vi "reward_behavior_michelle_visjitter_conswinAdapt_enticefx_TSLogV2.vi"() -> ()   [LabVIEW 2019]
doc: "The myRIO Project template acquires acceleration data from the onboard accelerometer and displays the changes of acceleration values in a waveform chart."
uses:
  <vilib>/myRIO/Common/Instrument Driver Framework/Utilities/typedefs/Generic FPGA Reference.ctl
  <vilib>/myRIO/Common/Instrument Driver Framework/Utilities/typedefs/myRIO v1.0 Reference.ctl
  <vilib>/myRIO/Common/Instrument Driver Framework/Utilities/typedefs/Hardware Version Enum.ctl
  <vilib>/myRIO/Common/Instrument Driver Framework/Utilities/typedefs/myRIO Generic Hardware Reference.ctl
  <vilib>/userdefined/High Color/nirio_resource_hc.ctl
  <vilib>/myRIO/Common/Instrument Driver Framework/Utilities/vis/Is FPGA Ref Available.vi
  <vilib>/myRIO/Common/Instrument Driver Framework/myRIO v1.0/Encoder/typedefs/Encoder Signal Mode.ctl
  <vilib>/myRIO/Common/Instrument Driver Framework/myRIO v1.0/Encoder/typedefs/Encoder Channels Enum.ctl
  <vilib>/myRIO/Instrument Drivers/Onboard IO/Encoder/typedefs/Encoder Reference.ctl
  <vilib>/myRIO/Instrument Drivers/Onboard IO/Encoder/Encoder.lvlib
  <vilib>/myRIO/Instrument Drivers/Onboard IO/Encoder/vis/Read.vi
  <vilib>/myRIO/Common/Instrument Driver Framework/myRIO v1.0/Encoder/typedefs/Encoder Configuration v1.0.ctl
  <vilib>/myRIO/Common/Instrument Driver Framework/myRIO v1.0/Encoder/vis/myRIO v1.1 Open Encoder.vi
  <vilib>/myRIO/Common/Instrument Driver Framework/myRIO v1.0/Encoder/vis/myRIO v1.0 Configure Encoder.vi
  <vilib>/myRIO/Instrument Drivers/Onboard IO/Encoder/vis/myRIO Encoder Open.xnode
  <vilib>/myRIO/Express VI/Onboard IO/Encoder/Encoder Express VI.xnode
  <vilib>/myRIO/Express VI/Onboard IO/DI/DI Express VI.xnode
  <vilib>/myRIO/Instrument Drivers/Onboard IO/DIO/vis/Read.vi
  <vilib>/myRIO/Instrument Drivers/Onboard IO/DIO/DIO.lvlib
  <vilib>/myRIO/Common/Instrument Driver Framework/myRIO v1.0/DIO/typedefs/DIO Channels Enum.ctl
  <vilib>/myRIO/Common/Instrument Driver Framework/myRIO v1.0/DIO/typedefs/DIO Channels List.ctl
  <vilib>/myRIO/Instrument Drivers/Onboard IO/DIO/typedefs/DIO Reference.ctl
  <vilib>/myRIO/Instrument Drivers/Onboard IO/DIO/vis/myRIO DIO Open.xnode
  <vilib>/myRIO/Common/Instrument Driver Framework/myRIO v1.0/DIO/vis/myRIO v1.1 Open DIO.vi
  <vilib>/myRIO/Instrument Drivers/Onboard IO/DIO/vis/Write.vi
  <vilib>/myRIO/Express VI/Onboard IO/DO/DO Express VI.xnode
  <vilib>/Analysis/Matrix/Datatypes/RealMatrix.ctl
  <vilib>/Analysis/Matrix/NI_Matrix.lvlib
panel:
  out "TimeLag":dbl
  out "Lag2":dbl
  out "TestTime":dbl
  out "RewTS":dbl[][](array[numeric])
  out "ConsTS":dbl[][](array[numeric])
  out "LickTS":dbl[][](array[numeric])
  out "ContrastChoice":dbl
  out "Its":i32
  out "BurstCriteria":dbl
  out "LickBurst 2":bool
  out "LickBurst":bool
  out "Enticements":i32
  in  "Entice":bool
  out "Misses":i32
  out "GoAhead":bool
  out "TimeOutDuration":i32
  out "ActiveTime":dbl
  out "ConsumptionGo":bool=TRUE
  out "Consumption_Period":i32
  out "Watch_Display":bool=TRUE
  in  "Give reward":bool
  out "Timings":dbl[](array[numeric])
  out "ISI":dbl
  out "ISI start time":dbl
  out "Time_out":bool=TRUE
  out "Time since lick":dbl
  out "Time of last lick":dbl
  out "Rewarded trials":dbl[](array[numeric])
  out "Rewards":u16
  out "Active Trial":bool
  out "Array temp2":T1
  out "Stimuli Loaded":bool
  out "Stim_ID":dbl[](array[numeric])
  out "Reward_mat":dbl[](array[numeric])
  out "Reward":bool=TRUE
  out "Frame clock":i32
  out "Licks":u32
  out "Lick":bool
  out "Time":dbl
  out "Stop":bool
  in  "Frames to collect":u32
  out "Overflow?":bool
  out "Counter Value":i32
  out "Velocity":dbl
  out "Velocity Plot":dbl[](graph)
  out "Velocity array":dbl[](array[numeric])
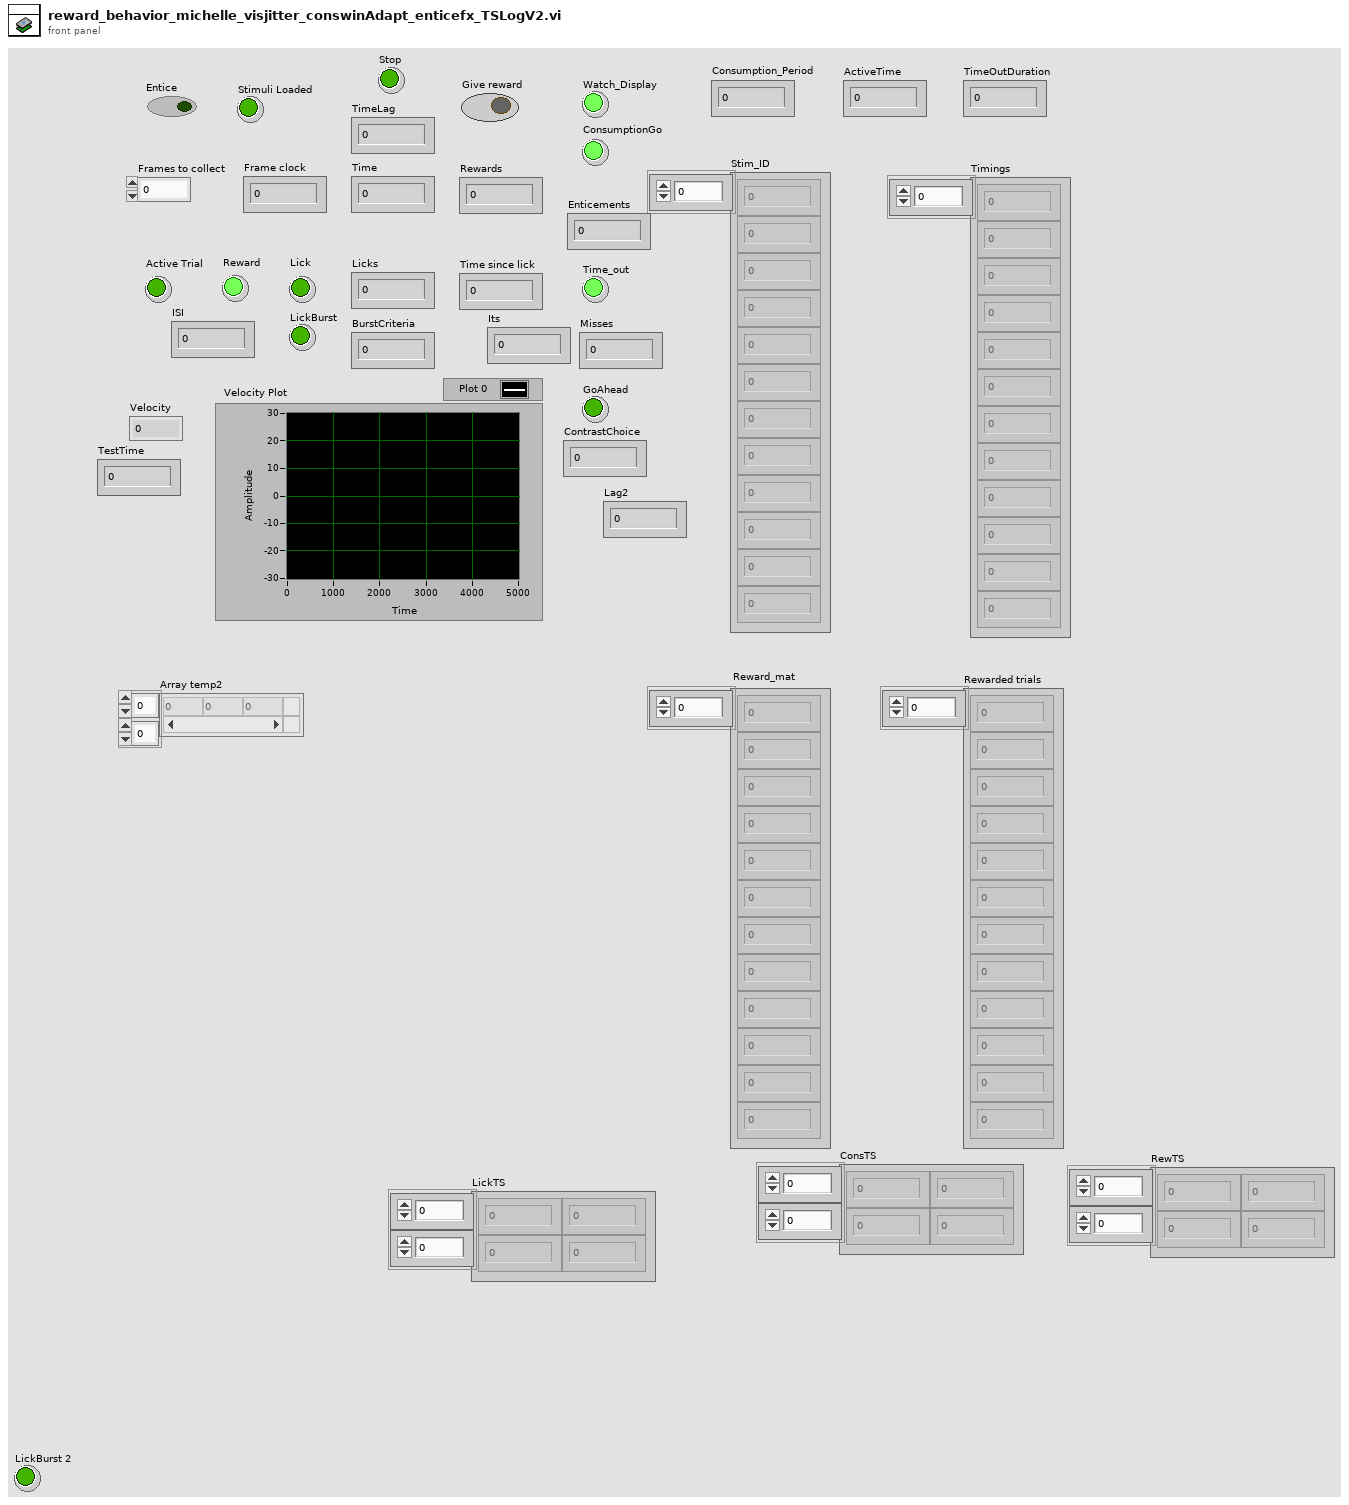
[diagram p1: front panel]
types:
  T1 = typedef "NI_Matrix.lvlib/RealMatrix.ctl" = dbl[][]
  T2 = typedef "Encoder.lvlib/Encoder Reference.ctl" = cluster{"myRIO Reference":T3, "Encoder Channels Enum":T7}
  T3 = typedef "myRIO Generic Hardware Reference.ctl" = cluster{"myRIO Model":T4, "myRIO Hardware Reference":T5}
  T4 = typedef "Hardware Version Enum.ctl" = enum16{"Unknown", "myRIO-1900", "myRIO-1950", "roboRIO", "NI ELVIS RIO CM", "ELVIS III"}
  T5 = typedef "myRIO v1.0 Reference.ctl" = cluster{"Generic FPGA Reference":T6, "Allow multiple opens":bool}
  T6 = typedef "Generic FPGA Reference.ctl" = refnum<k20>
  T7 = typedef "Encoder Channels Enum.ctl" = enum16{"Not Connected", "C/ENC0", "C/ENC1", "A/ENC", "A/ENC0", "A/ENC1", "A/ENC2", "A/ENC3", "A/ENC4", "A/ENC5", "A/ENC6", "A/ENC7", "A/ENC8", "A/ENC9", "B/ENC", "B/ENC0", "B/ENC1", "B/ENC2", "B/ENC3", "B/ENC4", "B/ENC5", "B/ENC6", "B/ENC7", "B/ENC8", "B/ENC9", "DIO/ENC0", "DIO/ENC1", "DIO/ENC2", "DIO/ENC3", "DIO/ENC4"}
  T8 = typedef "Encoder Signal Mode.ctl" = enum16{"Quadrature phase signal", "Step and direction signal"}
  T9 = typedef "nirio_resource_hc.ctl" = tag
  T10 = typedef "DIO.lvlib/DIO Reference.ctl" = cluster{"myRIO Reference":T3, "DIO Channels List":T11}
  T11 = typedef "DIO Channels List.ctl" = T12[]
  T12 = typedef "DIO Channels Enum.ctl" = enum16{"Not Connected", "C/DIO0", "C/DIO1", "C/DIO2", "C/DIO3", "C/DIO4", "C/DIO5", "C/DIO6", "C/DIO7", "A/DIO0", "A/DIO1", "A/DIO2", "A/DIO3", "A/DIO4", "A/DIO5", "A/DIO6", "A/DIO7", "A/DIO8", "A/DIO9", "A/DIO10", "A/DIO11", "A/DIO12", "A/DIO13", "A/DIO14", "A/DIO15", "A/DIO16", "A/DIO17", "A/DIO18", "A/DIO19", "B/DIO0", "B/DIO1", "B/DIO2", "B/DIO3", "B/DIO4", "B/DIO5", "B/DIO6", "B/DIO7", "B/DIO8", "B/DIO9", "B/DIO10", "B/DIO11", "B/DIO12", "B/DIO13", "B/DIO14", "B/DIO15", "B/DIO16", "B/DIO17", "B/DIO18", "B/DIO19", "LED0", "LED1", "LED2", "LED3", "Button0", "DIO/DIO0", "DIO/DIO1", "DIO/DIO2", "DIO/DIO3", "DIO/DIO4", "DIO/DIO5", "DIO/DIO6", "DIO/DIO7", "DIO/DIO8", "DIO/DIO9", "SPI/CS0", "SPI/CS1", "SPI/CS2", "SPI/CS3", "LED RADIO (Green)", "LED RADIO (Red)", "LED COMM (Green)", "LED COMM (Red)", "LED MODE (Green)", "LED MODE (Red)"}
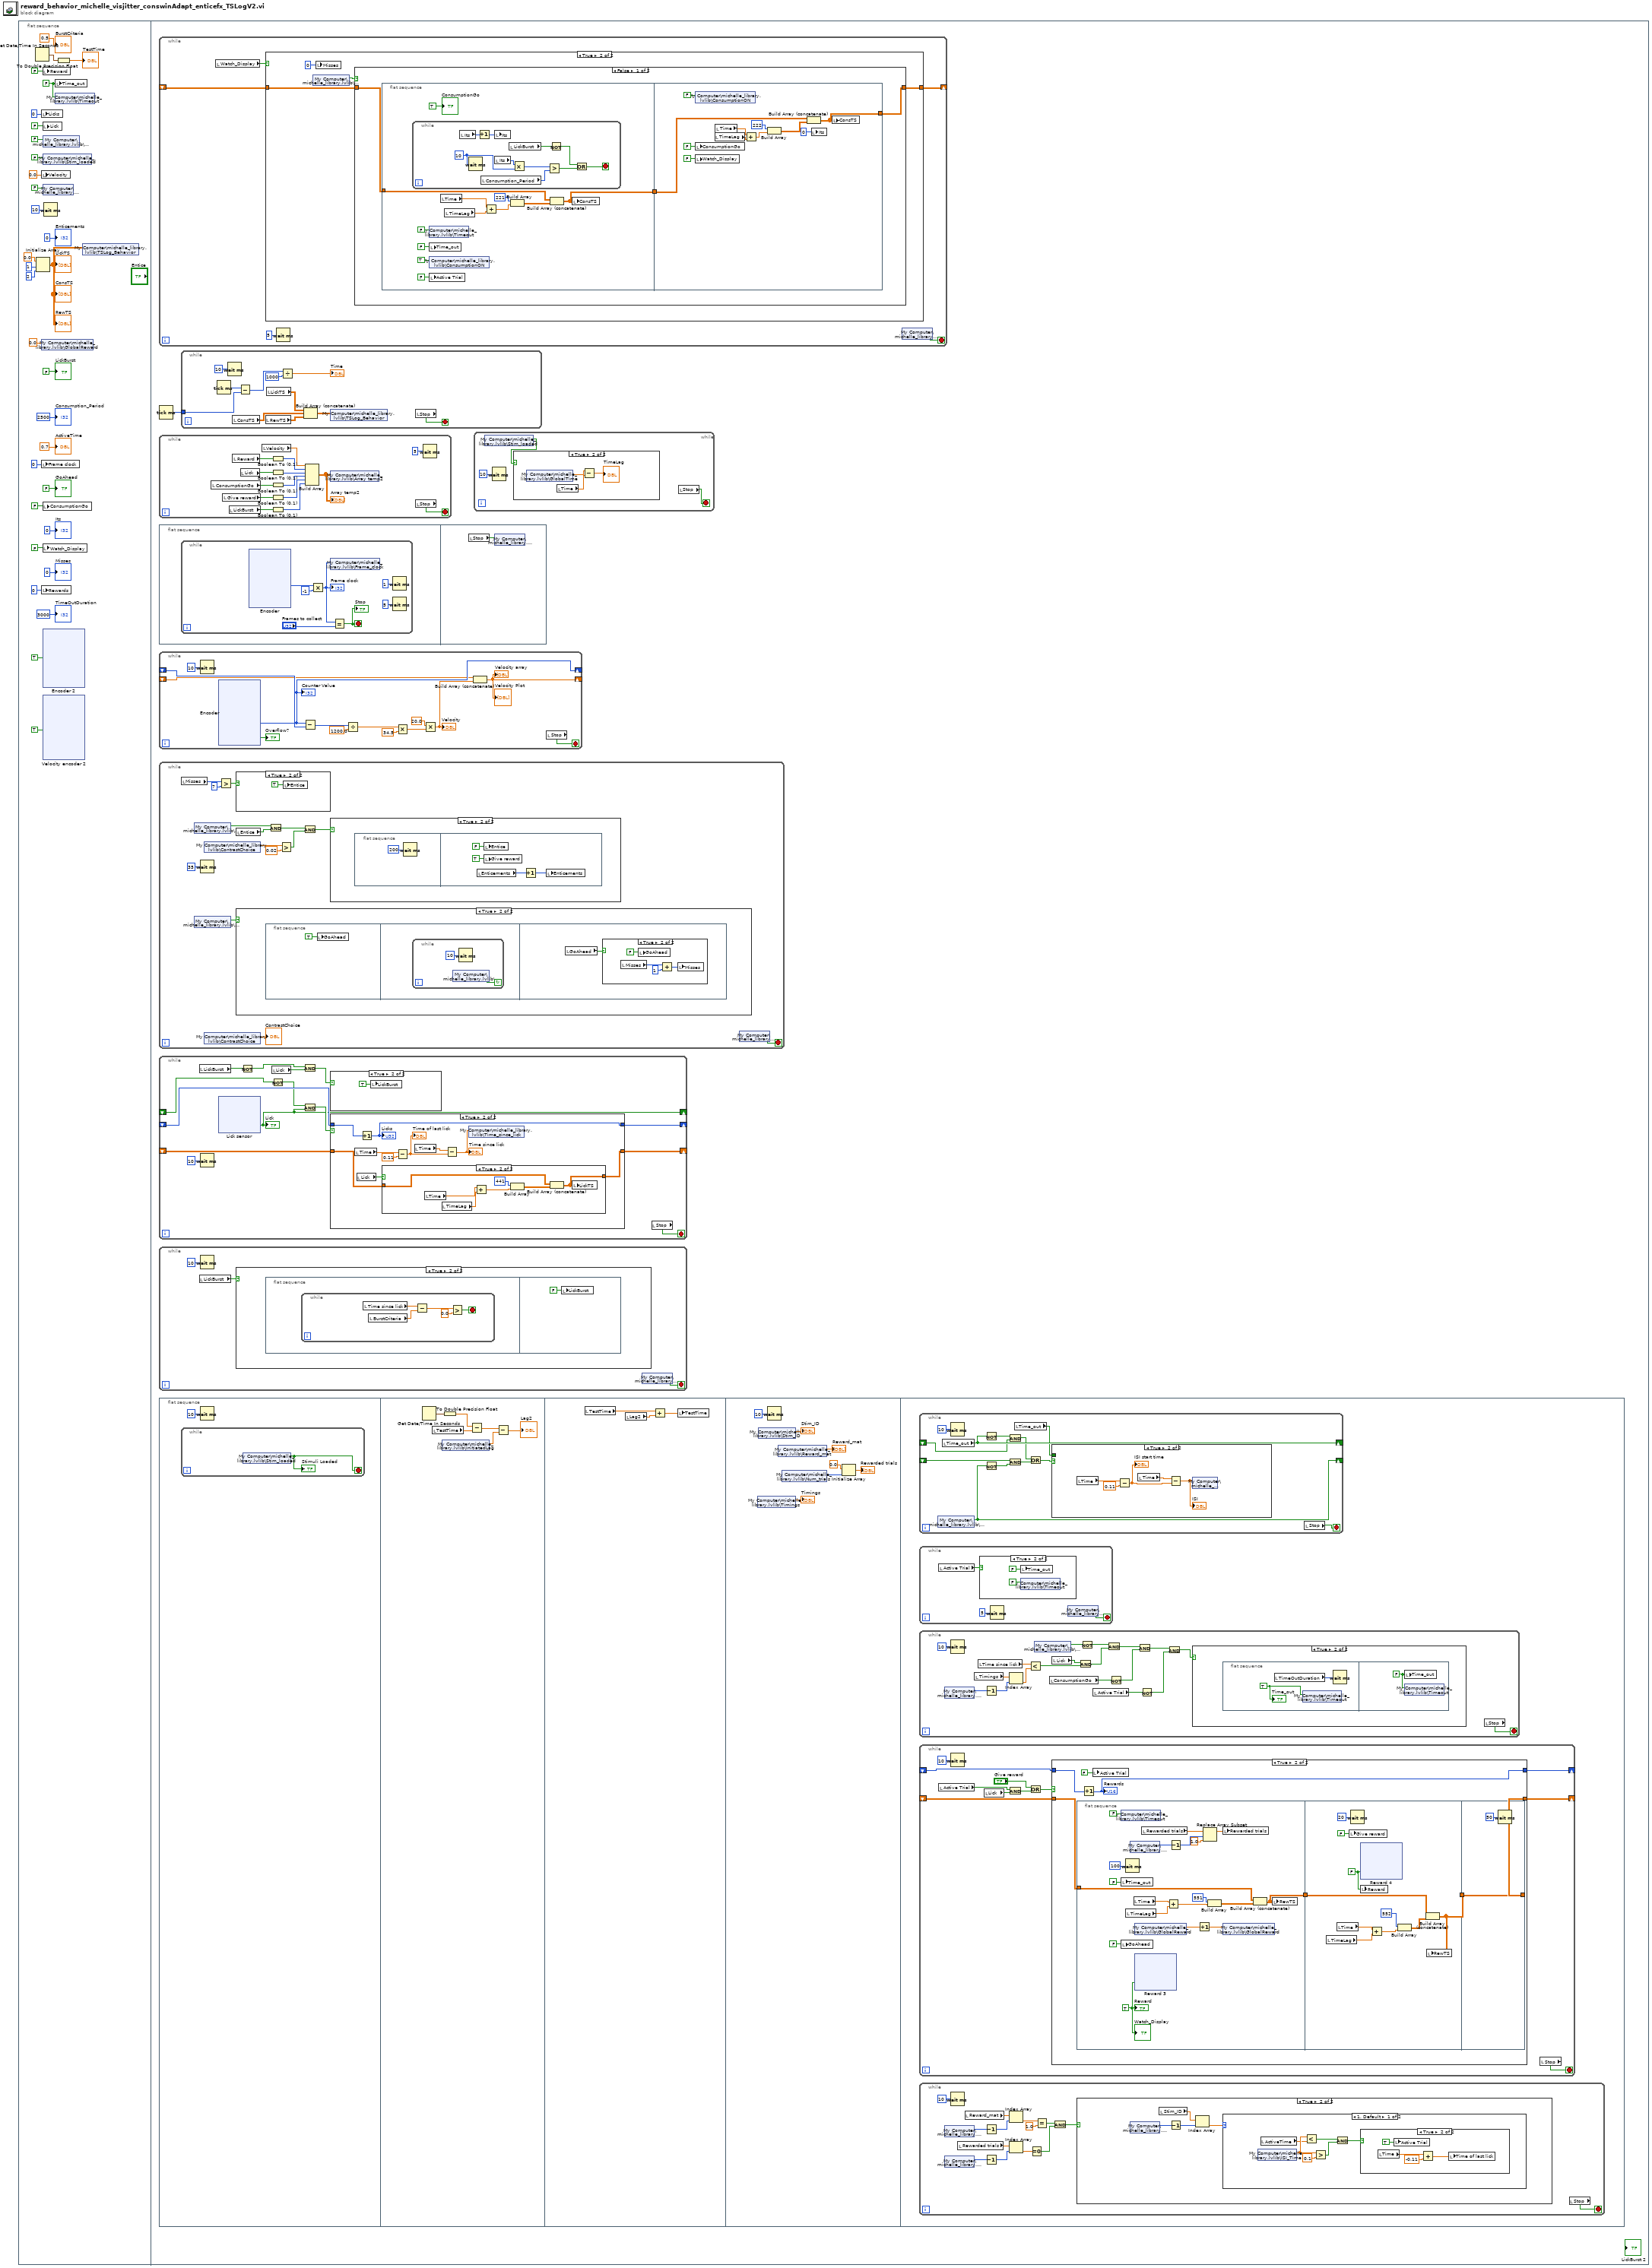
[diagram p0: block diagram]
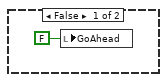
[diagram p6: hidden frame]
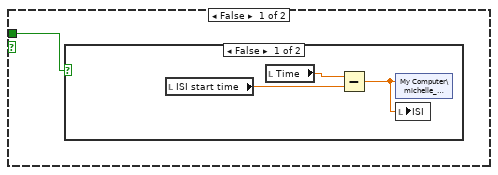
[diagram p12: hidden frame]
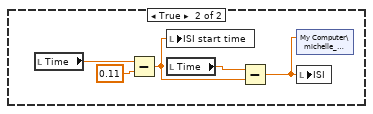
[diagram p13: hidden frame]
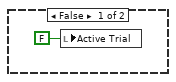
[diagram p14: hidden frame]
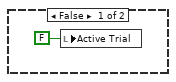
[diagram p15: hidden frame]
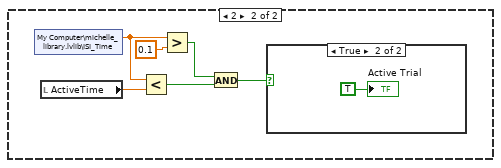
[diagram p16: hidden frame]
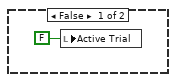
[diagram p17: hidden frame]
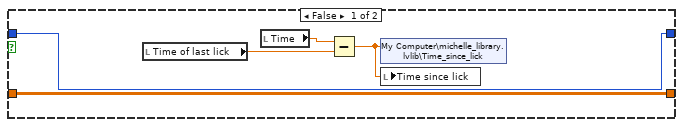
[diagram p20: hidden frame]
diagram:
  n1 = flat-sequence {
    frame #0 {
      w19 = FALSE ("Time_out")
      n2 = Get Date/Time In Seconds() -> (seconds since 1Jan1904=w3:timestamp)
      n3 = Initialize Array(0.0, 1, 2) -> (w1:dbl[][])
      "LickTS" <- w1
      "ConsTS" <- w1
      "RewTS" <- w1
      n4 = local write "Licks"(u32 0 ("Licks")) -> ()
      n5 = local write "Velocity"(0.0 ("Velocity")) -> ()
      n6 = shared-variable "My Computer\\michelle_library.lvlib\\GlobalReward"(0.0) -> ()  [unwired: 1 in, 1 out]
      n7 = local write "Frame clock"(u32 0 ("Frames")) -> ()
      n8 = local write "Rewards"(u16 0 ("Rewards")) -> ()
      n9 = local write "Reward"(FALSE ("Give reward")) -> ()
      n10 = local write "Lick"(FALSE ("Lick")) -> ()
      n11 = shared-variable "My Computer\\michelle_library.lvlib\\Display"(FALSE ("Display")) -> ()  [unwired: 1 in, 1 out]
      n12 = shared-variable "My Computer\\michelle_library.lvlib\\Stim_loaded"(FALSE ("Stim_loaded")) -> ()  [unwired: 1 in, 1 out]
      n13 = shared-variable "My Computer\\michelle_library.lvlib\\Stop"(FALSE ("Stop")) -> ()  [unwired: 1 in, 1 out]
      n14 = local write "ConsumptionGo"(FALSE ("ConsumptionGo")) -> ()
      n15 = local write "Watch_Display"(FALSE ("Watch_Display")) -> ()
      n16 = xnode "Encoder 2"("Reset Counter"=TRUE) -> ()  [unwired: 1 in, 4 out]
      n17 = xnode "Velocity encoder 2"("Reset Counter"=TRUE) -> ()  [unwired: 1 in, 4 out]
      n18 = Wait (ms)(milliseconds to wait=u32 10) -> ()  [unwired: 1 out]
      n19 = local write "Time_out"(w19) -> ()
      n20 = shared-variable "My Computer\\michelle_library.lvlib\\Timeout"(w19) -> ()  [unwired: 1 in, 1 out]
      n21 = To Double Precision Float(number=w3) -> (double precision float=→"TestTime":dbl)
      n22 = shared-variable "My Computer\\michelle_library.lvlib\\TSLog_Behavior"(w1) -> ()  [unwired: 1 in, 1 out]
      "Consumption_Period" <- 2500
      "ActiveTime" <- 0.7
      "TimeOutDuration" <- 3000
      "GoAhead" <- FALSE
      "Misses" <- 0
      "Enticements" <- 0
      "LickBurst" <- FALSE
      "BurstCriteria" <- 0.5
      "Its" <- 0
    }
    frame #1 {
      n23 = while {
        shift-right: [w169] -> _
        shift-left: _ -> [w170]
        stop <- w173 stop-if-true
        n24 = local read "Watch_Display"() -> (w172:bool)
        n25 = case shown="True" w172 {
          tunnel: w170 -> [w174 w176]
          tunnel: [w174 w175] -> w169
          frame False {
          }
          frame True {
            n26 = shared-variable "My Computer\\michelle_library.lvlib\\Display"() -> (w178:bool)  [unwired: 1 in, 1 out]
            n27 = local write "Misses"(0) -> ()
            n28 = case shown="False" w178 {
              tunnel: w176 -> [w181 w215]
              tunnel: [w179 w215] -> w175
              frame False {
                n29 = flat-sequence {
                  tunnel: w181 -> [w186]
                  tunnel: [w185] -> w180
                  tunnel: w180 -> [w209]
                  tunnel: [w208] -> w179
                  frame #0 {
                    n30 = while {
                      stop <- w197 stop-if-true
                      w198 = 10
                      n31 = local read "Its"() -> (w202:i32)
                      n32 = Wait (ms)(milliseconds to wait=w198) -> ()  [unwired: 1 out]
                      n33 = Increment(x=w202) -> (x+1=w201:i32)
                      n34 = local read "Consumption_Period"() -> (w195:i32)
                      n35 = local write "Its"(w201) -> ()
                      n36 = local read "Its"() -> (w199:i32)
                      n37 = local read "LickBurst"() -> (w203:bool)
                      n38 = Multiply(x=w199, y=w198) -> (x*y=w196:i32)
                      n39 = Greater?(x=w196, y=w195) -> (0:w194:bool)
                      n40 = Not(x=w203) -> (.not. x?=w200:bool)
                      n41 = Or(x=w200, y=w194) -> (x .or. y?=w197:bool)
                    }
                    n42 = shared-variable "My Computer\\michelle_library.lvlib\\Timeout"(FALSE) -> ()  [unwired: 1 in, 1 out]
                    n43 = local write "Time_out"(FALSE) -> ()
                    n44 = shared-variable "My Computer\\michelle_library.lvlib\\ConsumptionON"(TRUE) -> ()  [unwired: 1 in, 1 out]
                    n45 = local write "Active Trial"(FALSE) -> ()
                    n46 = local read "Time"() -> (w182:dbl)
                    n47 = local read "TimeLag"() -> (w183:dbl)
                    n48 = Add(x=w182, y=w183) -> (x+y=w184:dbl)
                    n49 = Build Array(221, w184) -> (w187:T1)
                    n50 = Build Array (concatenate) ("Build Matrix")(w186, w187) -> (w185:T1)
                    n51 = local write "ConsTS"(w185) -> ()
                    "ConsumptionGo" <- TRUE
                  }
                  frame #1 {
                    n52 = shared-variable "My Computer\\michelle_library.lvlib\\ConsumptionON"(FALSE) -> ()  [unwired: 1 in, 1 out]
                    n53 = local write "ConsumptionGo"(FALSE ("ConsumptionGo")) -> ()
                    n54 = local write "Watch_Display"(FALSE ("Watch_Display")) -> ()
                    n55 = local read "TimeLag"() -> (w205:dbl)
                    n56 = local read "Time"() -> (w204:dbl)
                    n57 = Add(x=w204, y=w205) -> (x+y=w206:dbl)
                    n58 = Build Array(222, w206) -> (w207:T1)
                    n59 = Build Array (concatenate) ("Build Matrix")(w209, w207) -> (w208:T1)
                    n60 = local write "Its"(0) -> ()
                    n61 = local write "ConsTS"(w208) -> ()
                  }
                }
              }
              frame True {
              }
            }
          }
        }
        n62 = Wait (ms)(milliseconds to wait=u32 5) -> ()  [unwired: 1 out]
        n63 = shared-variable "My Computer\\michelle_library.lvlib\\Stop"() -> (w173:bool)  [unwired: 1 in, 1 out]
      }
      n64 = Tick Count (ms)() -> (millisecond timer value=w124:u32)
      n65 = while {
        stop <- w223 stop-if-true
        n66 = local read "ConsumptionGo"() -> (w221:bool)
        n67 = local read "Give reward"() -> (w220:bool)
        n68 = local read "LickBurst"() -> (w217:bool)
        n69 = local read "Reward"() -> (w228:bool)
        n70 = local read "Lick"() -> (w229:bool)
        n71 = local read "Velocity"() -> (w227:dbl)
        n72 = Boolean To (0,1)(Boolean=w228) -> (0, 1=w226:i16)
        n73 = Boolean To (0,1)(Boolean=w229) -> (0, 1=w225:i16)
        n74 = Boolean To (0,1)(Boolean=w221) -> (0, 1=w219:i16)
        n75 = Boolean To (0,1)(Boolean=w220) -> (0, 1=w218:i16)
        n76 = Boolean To (0,1)(Boolean=w217) -> (0, 1=w216:i16)
        n77 = Build Array(w227, w226, w225, w219, w218, w216) -> (w222:T1)
        "Array temp2" <- w222
        n78 = shared-variable "My Computer\\michelle_library.lvlib\\Array temp2"(w222) -> ()  [unwired: 1 in, 1 out]
        n79 = local read "Stop"() -> (w223:bool)
        n80 = Wait (ms)(milliseconds to wait=u32 5) -> ()  [unwired: 1 out]
      }
      n81 = flat-sequence {
        frame #0 {
          n82 = while {
            stop <- w461 stop-if-true
            n83 = xnode "Encoder"() -> ("Counter Value"=w465:i32)  [unwired: 2 in, 3 out]
            n84 = Multiply(x=w465, y=-1) -> (x*y=w460:i32)
            "Frame clock" <- w460
            n85 = shared-variable "My Computer\\michelle_library.lvlib\\Frame_clock"(w460) -> ()  [unwired: 1 in, 1 out]
            n86 = Equal?(x=w460, y="Frames to collect") -> (x = y?=w461:bool)
            "Stop" <- w461
            n87 = Wait (ms)(milliseconds to wait=u32 1) -> ()  [unwired: 1 out]
            n88 = Wait (ms)(milliseconds to wait=u32 5) -> ()  [unwired: 1 out]
          }
        }
        frame #1 {
          n89 = local read "Stop"() -> (w513:bool)
          n90 = shared-variable "My Computer\\michelle_library.lvlib\\Stop"(w513) -> ()  [unwired: 1 in, 1 out]
        }
      }
      n91 = while {
        shift-right: [w597] -> _
        shift-left: _ -> [w598]
        shift-right: [w589] -> _
        shift-left: _ -> [w588]
        stop <- w587 stop-if-true
        n92 = Wait (ms)(milliseconds to wait=u32 10) -> ()  [unwired: 1 out]
        n93 = xnode "Encoder"() -> ("Counter Value"=w597:i32, "Overflow?"=→"Overflow?":bool)  [unwired: 2 in, 2 out]
        "Counter Value" <- w597
        n94 = Subtract(x=w597, y=w598) -> (x-y=w590:i32)
        n95 = Divide(x=w590, y=1200.0 ("600")) -> (x/y=w595:dbl)
        n96 = Multiply(x=w595, y=34.5) -> (x*y=w593:dbl)
        n97 = Multiply(x=20.0, y=w593) -> (x*y=w591:dbl)
        "Velocity" <- w591
        n98 = Build Array (concatenate)(w588, w591) -> (w589:dbl[])
        "Velocity Plot" <- w589
        "Velocity array" <- w589
        n99 = local read "Stop"() -> (w587:bool)
      }
      n100 = while {
        stop <- w153 stop-if-true
        n101 = local read "Misses"() -> (w151:i32)
        n102 = shared-variable "My Computer\\michelle_library.lvlib\\Display"() -> (w148:bool)  [unwired: 1 in, 1 out]
        n103 = shared-variable "My Computer\\michelle_library.lvlib\\Display"() -> (w152:bool)  [unwired: 1 in, 1 out]
        n104 = Wait (ms)(milliseconds to wait=35) -> ()  [unwired: 1 out]
        n105 = shared-variable "My Computer\\michelle_library.lvlib\\ContrastChoice"() -> (w144:dbl)  [unwired: 1 in, 1 out]
        n106 = shared-variable "My Computer\\michelle_library.lvlib\\ContrastChoice"() -> (→"ContrastChoice":dbl)  [unwired: 1 in, 1 out]
        n107 = Greater?(x=w151, y=7) -> (0:w149:bool)
        n108 = case shown="True" w149 {
          frame False {
          }
          frame True {
            n109 = local write "Entice"(TRUE) -> ()
          }
        }
        n110 = local read "Entice"() -> (w147:bool)
        n111 = case shown="True" w152 {
          frame False {
            n112 = local write "GoAhead"(FALSE) -> ()
          }
          frame True {
            n113 = flat-sequence {
              frame #0 {
                n114 = local write "GoAhead"(TRUE) -> ()
              }
              frame #1 {
                n115 = while {
                  stop <- w163 continue-if-true
                  n116 = shared-variable "My Computer\\michelle_library.lvlib\\Display"() -> (w163:bool)  [unwired: 1 in, 1 out]
                  n117 = Wait (ms)(milliseconds to wait=10) -> ()  [unwired: 1 out]
                }
              }
              frame #2 {
                n118 = local read "GoAhead"() -> (w164:bool)
                n119 = case shown="True" w164 {
                  frame False {
                  }
                  frame True {
                    n120 = local read "Misses"() -> (w168:i32)
                    n121 = local write "GoAhead"(FALSE) -> ()
                    n122 = Add(x=w168, y=1) -> (x+y=w166:i32)
                    n123 = local write "Misses"(w166) -> ()
                  }
                }
              }
            }
          }
        }
        n124 = And(x=w148, y=w147) -> (x .and. y?=w145:bool)
        n125 = Greater?(x=w144, y=0.02) -> (0:w143:bool)
        n126 = And(x=w145, y=w143) -> (x .and. y?=w142:bool)
        n127 = case shown="True" w142 {
          frame False {
          }
          frame True {
            n128 = flat-sequence {
              frame #0 {
                n129 = Wait (ms)(milliseconds to wait=200) -> ()  [unwired: 1 out]
              }
              frame #1 {
                n130 = local read "Enticements"() -> (w156:i32)
                n131 = local write "Entice"(FALSE) -> ()
                n132 = local write "Give reward"(TRUE) -> ()
                n133 = Increment(x=w156) -> (x+1=w155:i32)
                n134 = local write "Enticements"(w155) -> ()
              }
            }
          }
        }
        n135 = shared-variable "My Computer\\michelle_library.lvlib\\Stop"() -> (w153:bool)  [unwired: 1 in, 1 out]
      }
      n136 = while {
        shift-right: [w526] -> _
        shift-left: _ -> [w525]
        shift-right: [w520] -> _
        shift-left: _ -> [w523]
        shift-right: [w514] -> _
        shift-left: _ -> [w515]
        stop <- w524 stop-if-true
        n137 = local read "LickBurst"() -> (w517:bool)
        n138 = Wait (ms)(milliseconds to wait=u32 10) -> ()  [unwired: 1 out]
        n139 = xnode "Lick sensor"() -> ("C/DIO1 (DIO1)"=w520:bool)  [unwired: 1 in, 1 out]
        "Lick" <- w520
        n140 = Not(x=w517) -> (.not. x?=w516:bool)
        n141 = Not(x=w523) -> (.not. x?=w522:bool)
        n142 = local read "Lick"() -> (w518:bool)
        n143 = And(x=w516, y=w518) -> (x .and. y?=w519:bool)
        n144 = And(x=w522, y=w520) -> (x .and. y?=w521:bool)
        n145 = case shown="True" w519 {
          frame False {
          }
          frame True {
            n146 = local write "LickBurst"(TRUE) -> ()
          }
        }
        n147 = case shown="True" w521 {
          tunnel: [w533 w543] -> w526
          tunnel: w525 -> [w533 w542]
          tunnel: w515 -> [w529 w534]
          tunnel: [w529 w536] -> w514
          frame False {
            n148 = local read "Time of last lick"() -> (w531:dbl)
            n149 = local read "Time"() -> (w532:dbl)
            n150 = Subtract(x=w532, y=w531) -> (x-y=w530:dbl)
            n151 = shared-variable "My Computer\\michelle_library.lvlib\\Time_since_lick"(w530) -> ()  [unwired: 1 in, 1 out]
            n152 = local write "Time since lick"(w530) -> ()
          }
          frame True {
            n153 = local read "Time"() -> (w539:dbl)
            n154 = local read "Lick"() -> (w535:bool)
            n155 = Increment(x=w542) -> (x+1=w543:u32)
            "Licks" <- w543
            n156 = case shown="True" w535 {
              tunnel: w534 -> [w544 w549]
              tunnel: [w544 w548] -> w536
              frame False {
              }
              frame True {
                n157 = local read "Time"() -> (w546:dbl)
                n158 = local read "TimeLag"() -> (w547:dbl)
                n159 = Add(x=w546, y=w547) -> (x+y=w545:dbl)
                n160 = Build Array(441, w545) -> (w551:T1)
                n161 = Build Array (concatenate) ("Build Matrix")(w549, w551) -> (w548:T1)
                n162 = local write "LickTS"(w548) -> ()
              }
            }
            n163 = Subtract(x=w539, y=0.11) -> (x-y=w537:dbl)
            "Time of last lick" <- w537
            n164 = local read "Time"() -> (w541:dbl)
            n165 = Subtract(x=w541, y=w537) -> (x-y=w540:dbl)
            "Time since lick" <- w540
            n166 = shared-variable "My Computer\\michelle_library.lvlib\\Time_since_lick"(w540) -> ()  [unwired: 1 in, 1 out]
          }
        }
        n167 = local read "Stop"() -> (w524:bool)
      }
      n168 = while {
        stop <- w133 stop-if-true
        n169 = local read "LickBurst"() -> (w131:bool)
        n170 = Wait (ms)(milliseconds to wait=u32 10) -> ()  [unwired: 1 out]
        n171 = case shown="True" w131 {
          frame False {
          }
          frame True {
            n172 = flat-sequence {
              frame #0 {
                n173 = while {
                  stop <- w136 stop-if-true
                  n174 = local read "Time since lick"() -> (w137:dbl)
                  n175 = local read "BurstCriteria"() -> (w138:dbl)
                  n176 = Subtract(x=w137, y=w138) -> (x-y=w134:dbl)
                  n177 = Greater?(x=w134, y=0.0) -> (0:w136:bool)
                }
              }
              frame #1 {
                n178 = local write "LickBurst"(FALSE) -> ()
              }
            }
          }
        }
        n179 = shared-variable "My Computer\\michelle_library.lvlib\\Stop"() -> (w133:bool)  [unwired: 1 in, 1 out]
      }
      n180 = flat-sequence {
        frame #0 {
          n181 = while {
            stop <- w231 stop-if-true
            n182 = shared-variable "My Computer\\michelle_library.lvlib\\Stim_loaded"() -> (w231:bool)  [unwired: 1 in, 1 out]
            "Stimuli Loaded" <- w231
          }
          n183 = Wait (ms)(milliseconds to wait=u32 10) -> ()  [unwired: 1 out]
        }
        frame #1 {
          n184 = Get Date/Time In Seconds() -> (seconds since 1Jan1904=w237:timestamp)
          n185 = local read "TestTime"() -> (w236:dbl)
          n186 = shared-variable "My Computer\\michelle_library.lvlib\\InitiatedLag"() -> (w234:dbl)  [unwired: 1 in, 1 out]
          n187 = To Double Precision Float(number=w237) -> (double precision float=w235:dbl)
          n188 = Subtract(x=w235, y=w236) -> (x-y=w232:dbl)
          n189 = Subtract(x=w232, y=w234) -> (x-y=→"Lag2":dbl)
        }
        frame #2 {
          n190 = local read "TestTime"() -> (w238:dbl)
          n191 = local read "Lag2"() -> (w239:dbl)
          n192 = Add(x=w238, y=w239) -> (x+y=w240:dbl)
          n193 = local write "TestTime"(w240) -> ()
        }
        frame #3 {
          n194 = shared-variable "My Computer\\michelle_library.lvlib\\Timings"() -> (→"Timings":dbl[])  [unwired: 1 in, 1 out]
          n195 = shared-variable "My Computer\\michelle_library.lvlib\\Stim_ID"() -> (→"Stim_ID":dbl[])  [unwired: 1 in, 1 out]
          n196 = Wait (ms)(milliseconds to wait=u32 10) -> ()  [unwired: 1 out]
          n197 = shared-variable "My Computer\\michelle_library.lvlib\\Reward_mat"() -> (→"Reward_mat":dbl[])  [unwired: 1 in, 1 out]
          n198 = shared-variable "My Computer\\michelle_library.lvlib\\Num_trials"() -> (w244:u32)  [unwired: 1 in, 1 out]
          n199 = Initialize Array(0.0 ("element"), w244) -> (→"Rewarded trials":dbl[])
        }
        frame #4 {
          n200 = while {
            shift-right: [w285] -> _
            shift-left: _ -> [w283]
            shift-right: [w281] -> _
            shift-left: _ -> [w280]
            stop <- w286 stop-if-true
            n201 = shared-variable "My Computer\\michelle_library.lvlib\\Display"() -> (w281:bool)  [unwired: 1 in, 1 out]
            n202 = local read "Time_out"() -> (w285:bool)
            n203 = Wait (ms)(milliseconds to wait=u32 10) -> ()  [unwired: 1 out]
            n204 = Not(x=w285) -> (.not. x?=w284:bool)
            n205 = Not(x=w281) -> (.not. x?=w279:bool)
            n206 = And(x=w284, y=w283) -> (x .and. y?=w278:bool)
            n207 = And(x=w280, y=w279) -> (x .and. y?=w277:bool)
            n208 = local read "Time_out"() -> (w282:bool)
            n209 = Or(x=w278, y=w277) -> (x .or. y?=w276:bool)
            n210 = case shown="True" w276 {
              tunnel: w282 -> [w287 _]
              frame False {
                n211 = case shown="False" w287 {
                  frame False {
                    n212 = local read "ISI start time"() -> (w290:dbl)
                    n213 = local read "Time"() -> (w289:dbl)
                    n214 = Subtract(x=w289, y=w290) -> (x-y=w288:dbl)
                    n215 = shared-variable "My Computer\\michelle_library.lvlib\\ISI"(w288) -> ()  [unwired: 1 in, 1 out]
                    n216 = local write "ISI"(w288) -> ()
                  }
                  frame True {
                    n217 = local read "Time"() -> (w295:dbl)
                    n218 = Subtract(x=w295, y=0.11) -> (x-y=w292:dbl)
                    n219 = local write "ISI start time"(w292) -> ()
                    n220 = local read "Time"() -> (w293:dbl)
                    n221 = Subtract(x=w293, y=w292) -> (x-y=w291:dbl)
                    n222 = shared-variable "My Computer\\michelle_library.lvlib\\ISI"(w291) -> ()  [unwired: 1 in, 1 out]
                    n223 = local write "ISI"(w291) -> ()
                  }
                }
              }
              frame True {
                n224 = local read "Time"() -> (w300:dbl)
                n225 = Subtract(x=w300, y=0.11) -> (x-y=w297:dbl)
                "ISI start time" <- w297
                n226 = local read "Time"() -> (w298:dbl)
                n227 = Subtract(x=w298, y=w297) -> (x-y=w296:dbl)
                "ISI" <- w296
                n228 = shared-variable "My Computer\\michelle_library.lvlib\\ISI"(w296) -> ()  [unwired: 1 in, 1 out]
              }
            }
            n229 = local read "Stop"() -> (w286:bool)
          }
          n230 = while {
            stop <- w250 stop-if-true
            n231 = local read "Active Trial"() -> (w249:bool)
            n232 = case shown="True" w249 {
              frame False {
              }
              frame True {
                n233 = local write "Time_out"(FALSE) -> ()
                n234 = shared-variable "My Computer\\michelle_library.lvlib\\Timeout"(FALSE) -> ()  [unwired: 1 in, 1 out]
              }
            }
            n235 = Wait (ms)(milliseconds to wait=5) -> ()  [unwired: 1 out]
            n236 = shared-variable "My Computer\\michelle_library.lvlib\\Stop"() -> (w250:bool)  [unwired: 1 in, 1 out]
          }
          n237 = while {
            stop <- w271 stop-if-true
            n238 = shared-variable "My Computer\\michelle_library.lvlib\\Trial"() -> (w261:u32)  [unwired: 1 in, 1 out]
            n239 = Wait (ms)(milliseconds to wait=u32 10) -> ()  [unwired: 1 out]
            n240 = local read "Timings"() -> (w263:dbl[])
            n241 = local read "Time since lick"() -> (w270:dbl)
            n242 = Decrement(x=w261) -> (x-1=w260:u32)
            n243 = Index Array(array=w263, index=w260) -> (element=w262:dbl)
            n244 = Less?(x=w270, y=w262) -> (x < y?=w269:bool)
            n245 = shared-variable "My Computer\\michelle_library.lvlib\\Display"() -> (w266:bool)  [unwired: 1 in, 1 out]
            n246 = local read "ConsumptionGo"() -> (w258:bool)
            n247 = local read "Lick"() -> (w268:bool)
            n248 = And(x=w268, y=w269) -> (x .and. y?=w264:bool)
            n249 = Not(x=w266) -> (.not. x?=w265:bool)
            n250 = local read "Active Trial"() -> (w253:bool)
            n251 = And(x=w265, y=w264) -> (x .and. y?=w257:bool)
            n252 = Not(x=w258) -> (.not. x?=w259:bool)
            n253 = And(x=w257, y=w259) -> (x .and. y?=w255:bool)
            n254 = Not(x=w253) -> (.not. x?=w256:bool)
            n255 = And(x=w255, y=w256) -> (x .and. y?=w254:bool)
            n256 = case shown="True" w254 {
              frame False {
              }
              frame True {
                n257 = flat-sequence {
                  frame #0 {
                    w273 = TRUE
                    n258 = local read "TimeOutDuration"() -> (w272:i32)
                    n259 = shared-variable "My Computer\\michelle_library.lvlib\\Timeout"(w273) -> ()  [unwired: 1 in, 1 out]
                    n260 = Wait (ms)(milliseconds to wait=w272) -> ()  [unwired: 1 out]
                    "Time_out" <- w273
                  }
                  frame #1 {
                    w274 = FALSE ("Timeout")
                    n261 = local write "Time_out"(w274) -> ()
                    n262 = shared-variable "My Computer\\michelle_library.lvlib\\Timeout"(w274) -> ()  [unwired: 1 in, 1 out]
                  }
                }
              }
            }
            n263 = local read "Stop"() -> (w271:bool)
          }
          n264 = while {
            shift-right: [w347] -> _
            shift-left: _ -> [w346]
            shift-right: [w339] -> _
            shift-left: _ -> [w340]
            stop <- w349 stop-if-true
            n265 = local read "Active Trial"() -> (w344:bool)
            n266 = Wait (ms)(milliseconds to wait=u32 10) -> ()  [unwired: 1 out]
            n267 = local read "Lick"() -> (w345:bool)
            n268 = And(x=w344, y=w345) -> (x .and. y?=w343:bool)
            n269 = Or(x="Give reward", y=w343) -> (x .or. y?=w342:bool)
            n270 = case shown="True" w342 {
              tunnel: [w351 w358] -> w347
              tunnel: w346 -> [w351 w357]
              tunnel: w340 -> [w350 w355]
              tunnel: [w350 w354] -> w339
              frame False {
              }
              frame True {
                n271 = flat-sequence {
                  tunnel: w355 -> [w364]
                  tunnel: [w362] -> w352
                  tunnel: [w417] -> w353
                  tunnel: w352 -> [w416]
                  tunnel: [w458] -> w354
                  tunnel: w353 -> [w458]
                  frame #0 {
                    w376 = TRUE ("C/DIO0 (DIO0)")
                    n272 = shared-variable "My Computer\\michelle_library.lvlib\\Timeout"(FALSE) -> ()  [unwired: 1 in, 1 out]
                    n273 = local write "Time_out"(FALSE) -> ()
                    n274 = local write "GoAhead"(FALSE) -> ()
                    n275 = Wait (ms)(milliseconds to wait=u32 100) -> ()  [unwired: 1 out]
                    n276 = local read "TimeLag"() -> (w361:dbl)
                    n277 = shared-variable "My Computer\\michelle_library.lvlib\\Trial"() -> (w375:u32)  [unwired: 1 in, 1 out]
                    n278 = local read "Time"() -> (w360:dbl)
                    n279 = shared-variable "My Computer\\michelle_library.lvlib\\GlobalReward"() -> (w367:dbl)  [unwired: 1 in, 1 out]
                    n280 = xnode "Reward 3"("C/DIO0 (DIO0)"=w376) -> ()  [unwired: 1 in, 1 out]
                    n281 = local read "Rewarded trials"() -> (w373:dbl[])
                    n282 = Add(x=w360, y=w361) -> (x+y=w359:dbl)
                    n283 = Decrement(x=w375) -> (x-1=w374:u32)
                    n284 = Increment(x=w367) -> (x+1=w366:dbl)
                    n285 = Replace Array Subset(array=w373, new element=1.0 ("new element/subarray"), index=w374) -> (w371:dbl[])
                    n286 = Build Array(551, w359) -> (w365:T1)
                    n287 = local write "Rewarded trials"(w371) -> ()
                    n288 = shared-variable "My Computer\\michelle_library.lvlib\\GlobalReward"(w366) -> ()  [unwired: 1 in, 1 out]
                    n289 = Build Array (concatenate) ("Build Matrix")(w364, w365) -> (w362:T1)
                    n290 = local write "RewTS"(w362) -> ()
                    "Reward" <- w376
                    "Watch_Display" <- w376
                  }
                  frame #1 {
                    w422 = FALSE ("C/DIO0 (DIO0)")
                    n291 = local read "TimeLag"() -> (w413:dbl)
                    n292 = local read "Time"() -> (w414:dbl)
                    n293 = local write "Give reward"(FALSE ("Give reward")) -> ()
                    n294 = Wait (ms)(milliseconds to wait=u32 20) -> ()  [unwired: 1 out]
                    n295 = xnode "Reward 4"("C/DIO0 (DIO0)"=w422) -> ()  [unwired: 1 in, 1 out]
                    n296 = local write "Reward"(w422) -> ()
                    n297 = Add(x=w414, y=w413) -> (x+y=w415:dbl)
                    n298 = Build Array(552, w415) -> (w418:T1)
                    n299 = Build Array (concatenate) ("Build Matrix")(w416, w418) -> (w417:T1)
                    n300 = local write "RewTS"(w417) -> ()
                  }
                  frame #2 {
                    n301 = Wait (ms)(milliseconds to wait=u32 50) -> ()  [unwired: 1 out]
                  }
                }
                n302 = Increment(x=w357) -> (x+1=w358:u16)
                "Rewards" <- w358
                n303 = local write "Active Trial"(FALSE ("Active Trial")) -> ()
              }
            }
            n304 = local read "Stop"() -> (w349:bool)
          }
          n305 = while {
            stop <- w314 stop-if-true
            n306 = shared-variable "My Computer\\michelle_library.lvlib\\Trial"() -> (w310:u32)  [unwired: 1 in, 1 out]
            n307 = shared-variable "My Computer\\michelle_library.lvlib\\Trial"() -> (w306:u32)  [unwired: 1 in, 1 out]
            n308 = Wait (ms)(milliseconds to wait=u32 10) -> ()  [unwired: 1 out]
            n309 = local read "Rewarded trials"() -> (w307:dbl[])
            n310 = local read "Reward_mat"() -> (w309:dbl[])
            n311 = Decrement(x=w310) -> (x-1=w311:u32)
            n312 = Decrement(x=w306) -> (x-1=w305:u32)
            n313 = Index Array(array=w309, index=w311) -> (element=w312:dbl)
            n314 = Index Array(array=w307, index=w305) -> (element=w304:dbl)
            n315 = Equal To 0?(x=w304) -> (x = 0?=w303:bool)
            n316 = Equal?(x=w312, y=1.0) -> (x = y?=w302:bool)
            n317 = And(x=w302, y=w303) -> (x .and. y?=w301:bool)
            n318 = case shown="True" w301 {
              frame False {
                n319 = local write "Active Trial"(FALSE ("Active_trial")) -> ()
              }
              frame True {
                n320 = shared-variable "My Computer\\michelle_library.lvlib\\Trial"() -> (w317:u32)  [unwired: 1 in, 1 out]
                n321 = local read "Stim_ID"() -> (w319:dbl[])
                n322 = Decrement(x=w317) -> (x-1=w318:u32)
                n323 = Index Array(array=w319, index=w318) -> (element=w316:dbl)
                n324 = case shown="1, Default" w316 {
                  frame 1, Default {
                    n325 = shared-variable "My Computer\\michelle_library.lvlib\\ISI_Time"() -> (w325:dbl)  [unwired: 1 in, 1 out]
                    n326 = local read "ActiveTime"() -> (w320:dbl)
                    n327 = Less?(x=w325, y=w320) -> (x < y?=w323:bool)
                    n328 = Greater?(x=w325, y=0.1) -> (0:w322:bool)
                    n329 = And(x=w323, y=w322) -> (x .and. y?=w321:bool)
                    n330 = case shown="True" w321 {
                      frame False {
                        n331 = local write "Active Trial"(FALSE ("Active Trial")) -> ()
                      }
                      frame True {
                        n332 = local read "Time"() -> (w329:dbl)
                        n333 = local write "Active Trial"(TRUE ("Active Trial")) -> ()
                        n334 = Add(x=w329, y=-0.11) -> (x+y=w327:dbl)
                        n335 = local write "Time of last lick"(w327) -> ()
                      }
                    }
                  }
                  frame 2 {
                    n336 = shared-variable "My Computer\\michelle_library.lvlib\\ISI_Time"() -> (w335:dbl)  [unwired: 1 in, 1 out]
                    n337 = local read "ActiveTime"() -> (w331:dbl)
                    n338 = Less?(x=w335, y=w331) -> (x < y?=w333:bool)
                    n339 = Greater?(x=w335, y=0.1) -> (0:w334:bool)
                    n340 = And(x=w334, y=w333) -> (x .and. y?=w332:bool)
                    n341 = case shown="True" w332 {
                      frame False {
                        n342 = local write "Active Trial"(FALSE ("Active Trial")) -> ()
                      }
                      frame True {
                        "Active Trial" <- TRUE ("Active Trial")
                      }
                    }
                  }
                }
              }
            }
            n343 = local read "Stop"() -> (w314:bool)
          }
        }
      }
      n344 = while {
        tunnel: w124 -> [w656]
        stop <- w654 stop-if-true
        n345 = Tick Count (ms)() -> (millisecond timer value=w657:u32)
        n346 = Wait (ms)(milliseconds to wait=u32 10) -> ()  [unwired: 1 out]
        n347 = local read "ConsTS"() -> (w649:dbl[][])
        n348 = Subtract(x=w657, y=w656) -> (x-y=w653:u32)
        n349 = local read "RewTS"() -> (w648:dbl[][])
        n350 = local read "LickTS"() -> (w650:dbl[][])
        n351 = Divide(x=w653, y=u32 1000) -> (x/y=→"Time":dbl)
        n352 = Build Array (concatenate) ("Build Matrix")(w650, w649, w648) -> (w647:T1)
        n353 = shared-variable "My Computer\\michelle_library.lvlib\\TSLog_Behavior"(w647) -> ()  [unwired: 1 in, 1 out]
        n354 = local read "Stop"() -> (w654:bool)
      }
      n355 = while {
        stop <- w126 stop-if-true
        n356 = shared-variable "My Computer\\michelle_library.lvlib\\Stim_loaded"() -> (w127:bool)  [unwired: 1 in, 1 out]
        n357 = Wait (ms)(milliseconds to wait=u32 10) -> ()  [unwired: 1 out]
        n358 = case shown="True" w127 {
          frame False {
          }
          frame True {
            n359 = shared-variable "My Computer\\michelle_library.lvlib\\GlobalTime"() -> (w128:dbl)  [unwired: 1 in, 1 out]
            n360 = local read "Time"() -> (w129:dbl)
            n361 = Subtract(x=w128, y=w129) -> (x-y=→"TimeLag":dbl)
          }
        }
        n362 = local read "Stop"() -> (w126:bool)
      }
    }
  }
